vi "DownloadSpriteImages.vi"(8 "error in (no error)":errorcluster, 11 "Game in":refnum<class "Game.lvclass">) -> (0 "error out":errorcluster, 3 "Game out":refnum<class "Game.lvclass">)   [LabVIEW 2019, in "RT_Game.lvlib" / "Game.lvclass"]
uses:
  Game.lvclass
  Game.lvclass/Game.ctl
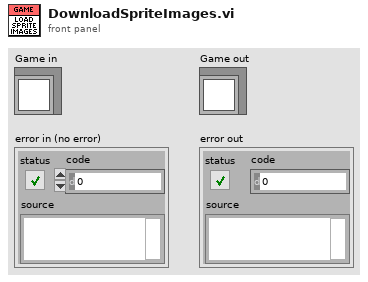
[diagram p1: front panel]
types:
  T1 = typedef "RT_Game.lvlib/Game.lvclass/SpritesCluster.ctl" = cluster{"Sprite1":refnum<class "RT_Sprite.lvclass">, "Sprite2":refnum<class "RT_Sprite.lvclass">, "Sprite3":refnum<class "RT_Sprite.lvclass">}
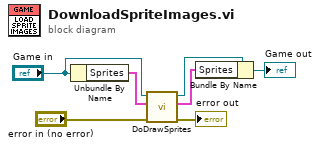
[diagram p0: block diagram]
diagram:
  n1 = Unbundle By Name("Game in") -> ("Sprites"=w4:T1)
  n2 = call "DoDrawSprites.vi"("error in (no error)"="error in (no error)", "Sprites in"=w4, "Game in"="Game in") -> ("error out"=→"error out":errorcluster, "Sprites out"=w6:T1, "Game out"=w7:refnum<class "Game.lvclass">)  [unwired: 6 in]
  n3 = Bundle By Name(cluster=w7, "Sprites"=w6) -> (→"Game out":refnum<class "Game.lvclass">)
